vi "DT3120_AsyncAquireFrame.vi"(8 "error in (no error)":errorcluster, 10 "Frame Size":T1, 11 "DevId":i32) -> (0 "error out":errorcluster, 2 "Frame":u32[][](array[numeric]), 3 "DevId (dup)":i32)   [LabVIEW 2009]
uses:
  olfg32.dll
panel:
  out "BytesWritten":u32
  out "BufSize":u32
  out "FrameId":u32
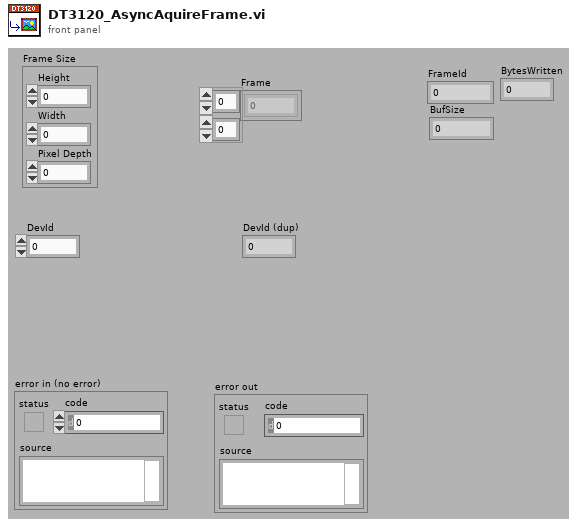
[diagram p1: front panel]
types:
  T1 = cluster{"Height":u32, "Width":u32, "Pixel Depth":u32}
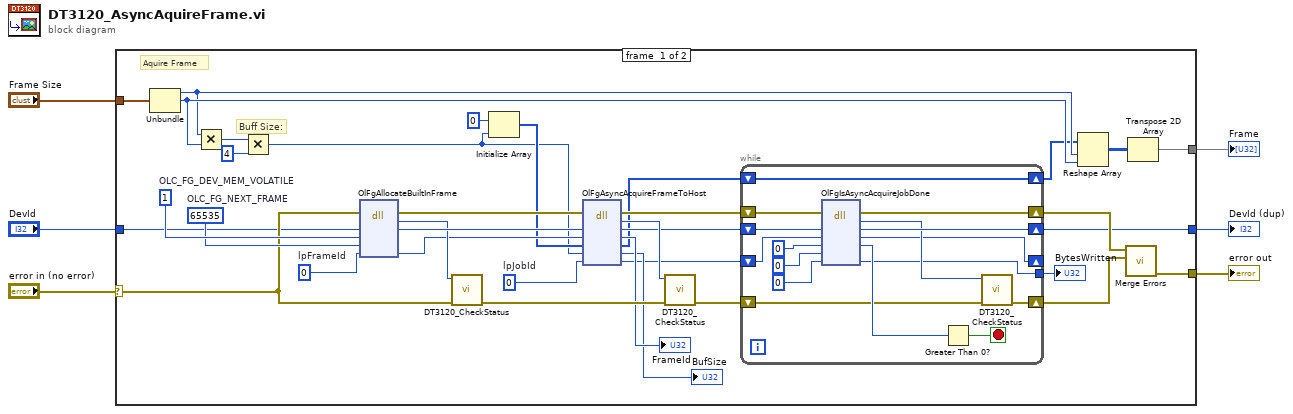
[diagram p0: block diagram]
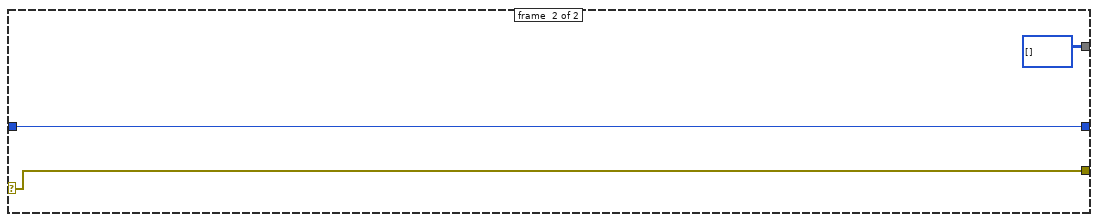
[diagram p2: hidden frame]
diagram:
  n1 = case shown="No Error" "error in (no error)" {
    selector: "error in (no error)" -> [w31 w60]
    tunnel: "DevId" -> [w30 w59]
    tunnel: [w39 w60] -> w5
    tunnel: [w11 w59] -> w4
    tunnel: "Frame Size" -> [w38 _]
    tunnel: [w21 u32[][] [] ("lpBuffer")] -> w1
    frame #0 {
      w17 = 0  # lpJobId
      w33 = u32 0  # lpFrameId
      w34 = u16 65535  # OLC_FG_NEXT_FRAME
      w35 = 1  # OLC_FG_DEV_MEM_VOLATILE
      # "Buff Size:"
      # "Aquire Frame"
      n2 = Unbundle(w38) -> ("Height"=w23:u32, "Width"=w24:u32)  [unwired: 1 out]
      n3 = Multiply(x=w23, y=w24) -> (x*y=w25:u32)
      n4 = Multiply(x=w25, y=u32 4) -> (x*y=w18:u32)
      n5 = dll-call lib="C:/LabVIEW Programs/MT Scan/SubVIs/olfg32.dll" fn="OlFgAllocateBuiltInFrame"(error in=w31, "DevId"=w30, "MemType"=w35, "BufNum"=w34, "lpFrameId"=w33) -> (error out=w32:errorcluster, "Status"=w28:u32, "DevId"=w29:i32, "lpFrameId"=w27:u32)  [unwired: 4 in, 1 out]
      n6 = call "DT3120_CheckStatus.vi"("error in"=w31, "Status"=w28) -> ("error out"=w41:errorcluster)  [unwired: 9 out]
      n7 = Initialize Array(u32 0 ("element"), w18) -> (w26:u32[])
      n8 = dll-call lib="C:/LabVIEW Programs/MT Scan/SubVIs/olfg32.dll" fn="OlFgAsyncAcquireFrameToHost"(error in=w32, "DevId"=w29, "FrameId"=w27, "lpBuffer"=w26, "BufSize"=w18, "lpJobId"=w17) -> (error out=w16:errorcluster, "Status"=w40:u32, "DevId"=w15:i32, "FrameId"=→"FrameId":u32, "lpBuffer"=w8:u32[], "BufSize"=→"BufSize":u32, "lpJobId"=w10:i32)  [unwired: 2 in, 1 out]
      n9 = call "DT3120_CheckStatus.vi"("error in"=w41, "Status"=w40) -> ("error out"=w14:errorcluster)  [unwired: 9 out]
      n10 = while {
        shift-right: [w53] -> w12
        shift-left: w16 -> [w57]
        shift-right: [w52] -> w11
        shift-left: w15 -> [w56]
        shift-right: [w49] -> w13
        shift-left: w14 -> [w51]
        shift-right: [w47] -> _
        shift-left: w10 -> [w48]
        tunnel: [w43] -> w9
        shift-right: [w42] -> w7
        shift-left: w8 -> [w42]
        stop <- w54 stop-if-true
        n11 = dll-call lib="C:/LabVIEW Programs/MT Scan/SubVIs/olfg32.dll" fn="OlFgIsAsyncAcquireJobDone"(error in=w57, "DevId"=w56, "JobId"=w48, "lpDone"=u8 0, "lpJobStatus"=0, "lpBytesWritten"=u32 0) -> (error out=w53:errorcluster, "Status"=w50:u32, "DevId"=w52:i32, "JobId"=w47:i32, "lpDone"=w55:u8, "lpBytesWritten"=w43:u32)  [unwired: 2 in, 2 out]
        n12 = Greater Than 0?(x=w55) -> (x > 0?=w54:bool)
        n13 = call "DT3120_CheckStatus.vi"("error in"=w51, "Status"=w50) -> ("error out"=w49:errorcluster)  [unwired: 9 out]
      }
      "BytesWritten" <- w9
      n14 = Reshape Array(w7, w23, w24) -> (w22:u32[][])
      n15 = call <vilib>:"Merge Errors.vi"("error in 2 (no error)"=w13, "error in 1 (no error)"=w12) -> ("error out"=w39:errorcluster)  [unwired: 2 in, 3 out]
      n16 = Transpose 2D Array(2D array=w22) -> (transposed array=w21:u32[][])
    }
    frame #1 {
    }
  }
  "error out" <- w5
  "DevId (dup)" <- w4
  "Frame" <- w1
